vi "Do.vi"(8 "error in (no error)":errorcluster, 10 "Actor in":refnum<class "Actor.lvclass">, 11 "Conceret Initialize Edit Project Msg in":refnum<class "Conceret Initialize Edit Project Msg.lvclass">) -> (0 "error out":errorcluster, 2 "Actor out":refnum<class "Actor.lvclass">)   [LabVIEW 2013, in "Edit Project View.lvlib" / "Conceret Initialize Edit Project Msg.lvclass"]
doc: "(<B>Filename</B>: Actor Framework.lvlib:Message.lvclass:Do.vi)\n\nDefines what a message does when it is received by an actor. Generally, a message instructs an actor to invoke one of its methods.\n\nBy default, this method does nothing. A child class must override it to define behavior. Create a child class by using the Actor Framework Message Maker dialog box."
uses:
  Conceret Initialize Edit Project Msg.lvclass
  <vilib>/ActorFramework/Actor/Actor.lvclass
  Edit Project View/Edit Project View.lvclass
  Models/Edit Project Model Messages/Abstract Initialize Edit Project Msg/Abstract Initialize Edit Project Msg.lvclass
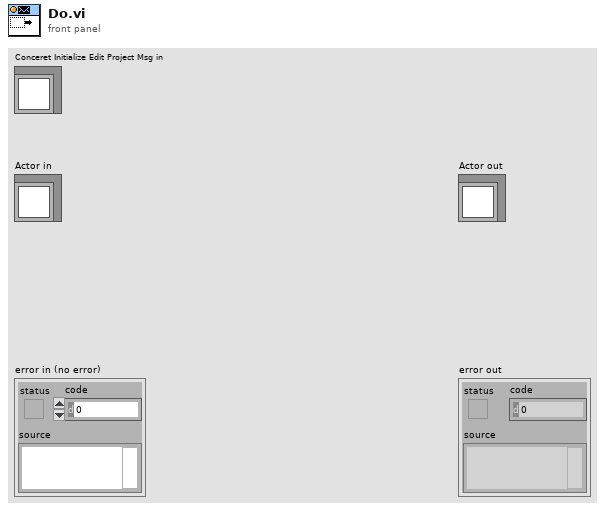
[diagram p1: front panel]
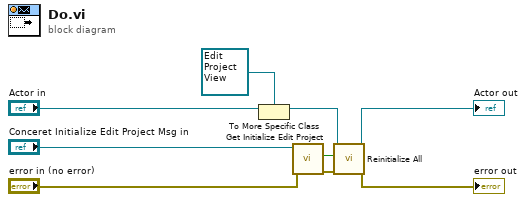
[diagram p0: block diagram]
diagram:
  n1 = To More Specific Class(target class=refnum<class "Edit Project View.lvclass"> refnum ("Edit Project View.lvlib:Edit Project View.lvclass"), reference="Actor in") -> (specific class reference=w6:refnum<class "Edit Project View.lvclass">)  [unwired: 1 in, 1 out]
  n2 = call "Get Initialize Edit Project.vi"("error in (no error)"="error in (no error)", "Abstract Initialize Edit Project Msg in"="Conceret Initialize Edit Project Msg in") -> ("error out"=w5:errorcluster, "Initialize Edit Project"=w1:bool)  [unwired: 7 in, 1 out]
  n3 = call "Reinitialize All.vi"("error in (no error)"=w5, "Initialize Edit Project"=w1, "Create Project View in"=w6) -> ("error out"=→"error out":errorcluster, "Create Project View out"=→"Actor out":refnum<class "Edit Project View.lvclass">)  [unwired: 7 in]
